vi "USB3 Upgrade Camera.vi"(8 "error in (no error)":errorcluster, 10 "pcPrivate":string, 11 "pcFw_UpgradeFileFullPath":string) -> (0 "error out":errorcluster, 3 "function return":i32)   [LabVIEW 2013, in "Octoplus_LIDAR.lvlib"]
doc: "CAMCMOSOCTUSB3_API int __cdecl USB3_UpgradeCamera(const char * pcFw_UpgradeFileFullPath, const char * pcPrivate);"
uses:
  <userlib>/Octoplus_LIDAR/Octoplus_LIDAR.lvlib
  <userlib>/Octoplus_LIDAR/CamCmosOctUsb3.dll
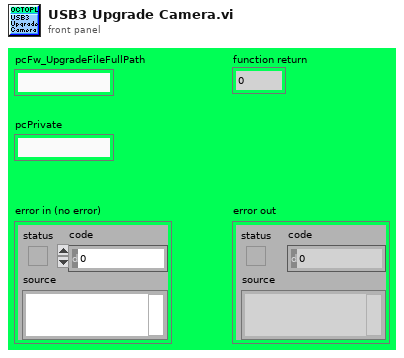
[diagram p1: front panel]
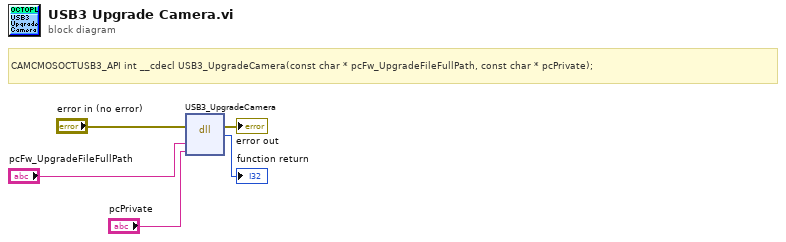
[diagram p0: block diagram]
diagram:
  # "CAMCMOSOCTUSB3_API int __cdecl USB3_UpgradeCamera(const char * pcFw_UpgradeFileFullPath, const char * pcPrivate);"
  n1 = dll-call lib="C:/Program Files/National Instruments/LabVIEW 2013/user.lib/Octoplus_LIDAR/CamCmosOctUsb3.*" fn="USB3_UpgradeCamera"(error in="error in (no error)", "pcFw_UpgradeFileFullPath"="pcFw_UpgradeFileFullPath", "pcPrivate"="pcPrivate") -> (error out=→"error out":errorcluster, →"function return":i32)  [unwired: 4 in, 1 out]
